vi "interpolate.vi"(8 "error in (no error)":errorcluster, 10 "element in":dbl, 11 "AOTF in":refnum<class "AOTF.lvclass">) -> (0 "error out":errorcluster, 2 "element out":dbl, 3 "AOTF out":refnum<class "AOTF.lvclass">)   [LabVIEW 2012, in "AOTF.lvclass"]
uses:
  AOTF.lvclass
  AOTF.lvclass/AOTF.ctl
  <vilib>/gmath/NI_Gmath.lvlib
panel:
  out "original graph":cluster{dbl[], "yi":dbl[]}(graph)
  out "transmitted":dbl[](array[numeric])
  out "AOTF power":dbl[](array[numeric])
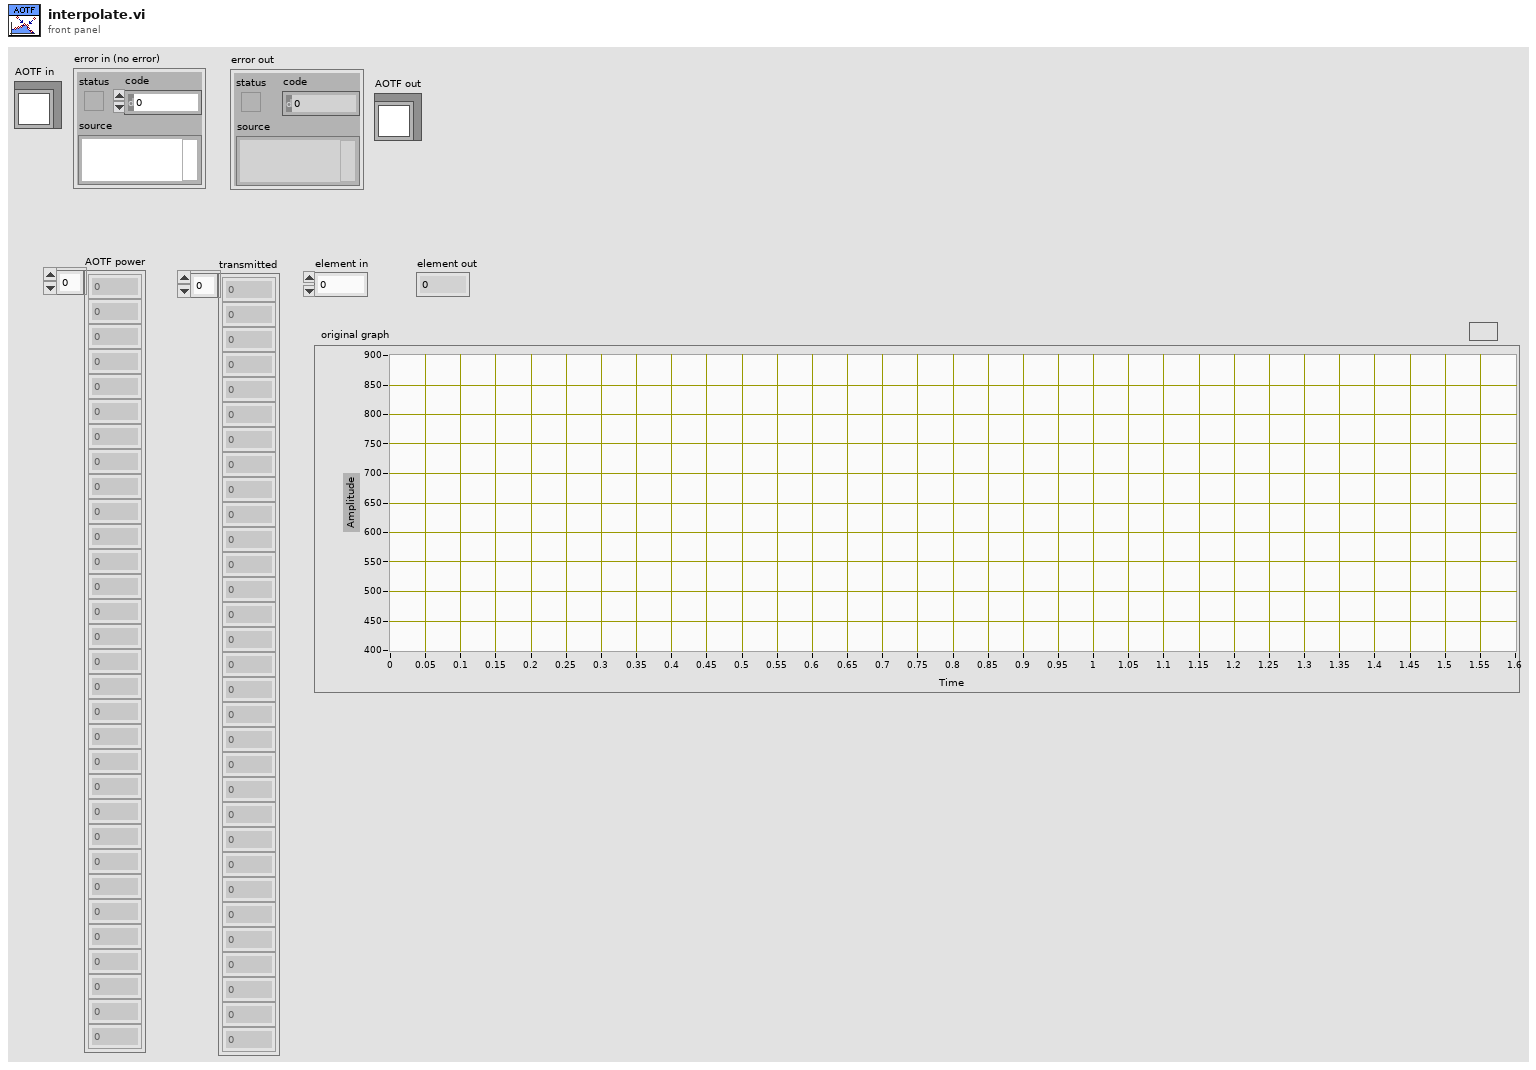
[diagram p1: front panel]
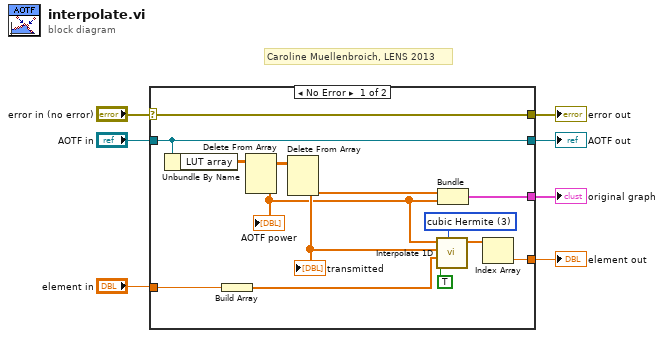
[diagram p0: block diagram]
diagram:
  # "Caroline Muellenbroich, LENS 2013"
  n1 = case shown="No Error" "error in (no error)" {
    selector: "error in (no error)" -> [w20 w22]
    tunnel: [w20 w22] -> w6
    tunnel: [w15 w21] -> w5
    tunnel: "AOTF in" -> [w15 w21]
    tunnel: [w16 _] -> w4
    tunnel: "element in" -> [w9 _]
    tunnel: [w8 _] -> w2
    frame No Error {
      w18 = 3 items=["nearest", "linear", "spline", "cubic Hermite", "Lagrange"] ("method")
      n2 = Unbundle By Name(w15) -> ("LUT array"=w14:dbl[][])
      n3 = Build Array(w9) -> (w11:dbl[])
      n4 = Delete From Array(array=w14) -> (deleted portion=w12:dbl[], array with subset deleted=w19:dbl[][])  [unwired: 3 in]
      "AOTF power" <- w12
      n5 = Delete From Array(array=w19) -> (deleted portion=w13:dbl[])  [unwired: 3 in, 1 out]
      "transmitted" <- w13
      n6 = call <vilib>:"Interpolate 1D.vi"("method"=w18, "X is monotonic"=TRUE, "xi"=w11, "X"=w13, "Y"=w12) -> ("yi"=w10:dbl[])  [unwired: 4 in, 2 out]
      n7 = Bundle("LUT array"=w13, "LUT array"=w12) -> (w16:cluster{"LUT array":dbl[], "LUT array":dbl[]})  [unwired: 1 in]
      n8 = Index Array(array=w10) -> (element=w8:dbl)  [unwired: 1 in]
    }
    frame Error {
    }
  }
  "error out" <- w6
  "AOTF out" <- w5
  "original graph" <- w4
  "element out" <- w2
